vi "sub CRC16_fery.vi"(6 "Data in":bool[](array[boolean])) -> (1 "Data + CRC 16":bool[](array[boolean]), 2 "CRC 16 out":bool[](array[boolean]))   [LabVIEW 2015]
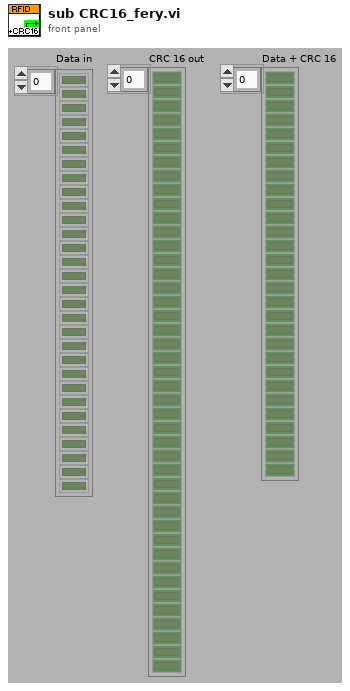
[diagram p1: front panel]
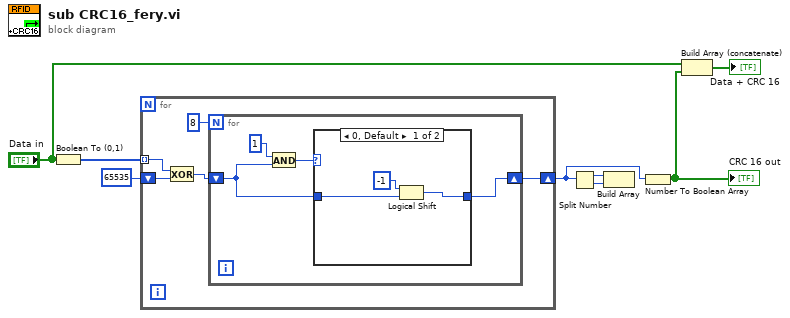
[diagram p0: block diagram]
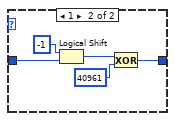
[diagram p2: hidden frame]
diagram:
  n1 = Boolean To (0,1)(Boolean="Data in") -> (0, 1=w1:i16[])
  n2 = for {
    shift-right: [w9] -> w4
    shift-left: 65535 -> [w12]
    tunnel: w1 -> [w11] mode=indexing
    n3 = Exclusive Or(1:w12, 2:w11) -> (0:w10:i32)
    n4 = for {
      N: 8 -> [_]
      shift-right: [w15] -> w9
      shift-left: w10 -> [w14]
      n5 = And(x=1, y=w14) -> (x .and. y?=w16:i32)
      n6 = case shown="0, Default" w16 {
        tunnel: w14 -> [w19 w21]
        tunnel: [w18 w25] -> w15
        frame 0, Default {
          n7 = Logical Shift(y=-1, x=w19) -> (x << y=w18:i32)
        }
        frame 1 {
          n8 = Logical Shift(y=-1, x=w21) -> (x << y=w22:i32)
          n9 = Exclusive Or(1:40961 ("y"), 2:w22) -> (0:w25:i32)
        }
      }
    }
  }
  n10 = Split Number(x=w4) -> (hi(x)=w8:u16, lo(x)=w7:u16)
  n11 = Build Array(w8, w7) -> ()  [unwired: 1 out]
  n12 = Number To Boolean Array(number=w4) -> (Boolean array=w5:bool[])
  "CRC 16 out" <- w5
  n13 = Build Array (concatenate)("Data in", w5) -> (→"Data + CRC 16":bool[])
